vi "XIPIN_Clocking_Wizard_5_2.vi"   [LabVIEW 2017]
doc: "The Clocking Wizard creates an HDL file (Verilog or VHDL) that contains a clocking circuit customized to the user's clocking requirements.\n------------------------------------\n<b>Need License</b> : No\n<b>Interface</b> : AXI4"
uses:
  <vilib>/rvi/XilinxIP/XIPIN_XNode/niFpgaXIPIN.xnode
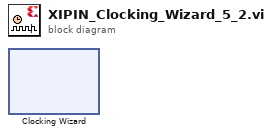
[diagram p0: block diagram]
diagram:
  n1 = xnode ("Clocking Wizard")() -> ()
